vi "ReplaceSelf.vi"(0 "XRef":T9, 1 "Terms":T6, 2 "Diagram":T5, 3 "State In":T4) -> (14 "Replace Self?":T1, 15 "Reply":T2)   [LabVIEW 2012, in "OpenG FilterArray.xnode"]
doc: "This ability VI is called when you want to replace this XNode via LabVIEW's scripting API. This VI is only called when you have previously informed LabVIEW that you want to replace the XNode through a ReplaceSelf reply. Diagram is a reference to a diagram of a temporary VI. This diagram contains exactly one front panel terminal for each terminal of your XNode. Terms is an array of pairs of Term IDs and terminal references. LabVIEW will replace your XNode with code scripted into this diagram into the diagram of the VI containing your XNode and connect everything to the correct terminals. The front panel terminals that are on this diagram are special in that they can only be on the top level diagram.\n \n Replace Self? is used to tell LabVIEW whether or not you want to copy the scripted diagram over. If there is an error and you wish not to commit the changes, then the old XNode behavior will be left unchanged. It will not be called again until you indicate that it should be through the reply on another ability VI.\n \n You should not use the Copy scripting method to move code into the temporary VI. This will adversely affect the user's clipboard. You should use the Move scripting method instead.\n\nDefault behavior: None.\n\nThis ability does not provide UI and OS messages are not handled.\n\nSee also: AugmentSelf"
uses:
  OpenG FilterArray.xnode
  <vilib>/XNodeSupport/XNodeXNodeRef.ctl
  <vilib>/XNodeSupport/XNodeTermIDPairs.ctl
  <vilib>/XNodeSupport/XNodeTermIDPair.ctl
  <vilib>/XNodeSupport/XNodeTermRef.ctl
  <vilib>/XNodeSupport/XNodeString.ctl
  <vilib>/XNodeSupport/XNodeTopLevelDiagramRef.ctl
  State.ctl
  <vilib>/XNodeSupport/XNodeStringArray.ctl
  <vilib>/XNodeSupport/XNodeBool.ctl
  <vilib>/Utility/miscctls.llb/LVPositionTypeDef.ctl
  <userlib>/_LAVAcr/Scripting Tools/Scripting Tools.lvlib
  <vilib>/XNodeSupport/NI_XNodeSupport.lvlib
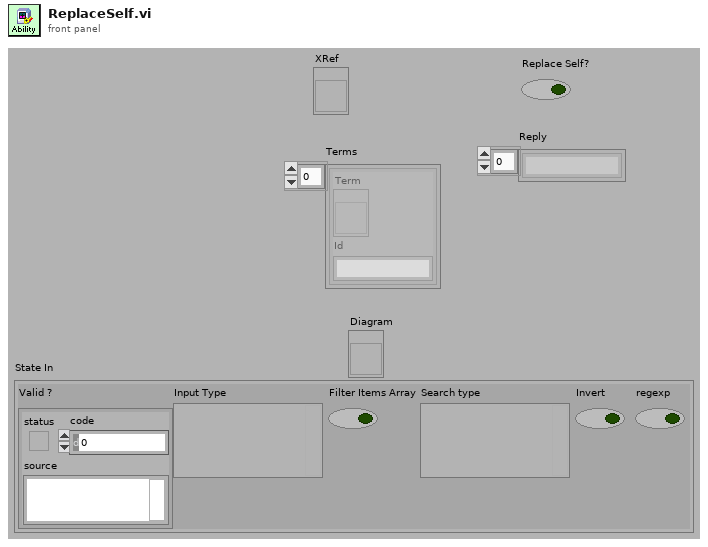
[diagram p1: front panel]
types:
  T1 = typedef "NI_XNodeSupport.lvlib/XNodeBool.ctl" = bool
  T2 = typedef "NI_XNodeSupport.lvlib/XNodeStringArray.ctl" = T3[]
  T3 = typedef "NI_XNodeSupport.lvlib/XNodeString.ctl" = string
  T4 = typedef "OpenG FilterArray.xnode/State.ctl" = cluster{"Valid ?":errorcluster, "Input Type":variant, "Filter Items Array":bool, "Search type":variant, "Invert":bool, "regexp":bool}
  T5 = typedef "NI_XNodeSupport.lvlib/XNodeTopLevelDiagramRef.ctl" = refnum<vi>
  T6 = typedef "NI_XNodeSupport.lvlib/XNodeTermIDPairs.ctl" = T7[]
  T7 = typedef "NI_XNodeSupport.lvlib/XNodeTermIDPair.ctl" = cluster{"Term":T8, "Id":T3}
  T8 = typedef "NI_XNodeSupport.lvlib/XNodeTermRef.ctl" = refnum<vi>
  T9 = typedef "NI_XNodeSupport.lvlib/XNodeXNodeRef.ctl" = refnum<vi>
  T10 = typedef "LVPositionTypeDef.ctl" = cluster{"Left":i32, "Top":i32}
  T11 = typedef "imagedata.ctl" = cluster{"image type":i32, "image depth":i32, "image":u8[], "mask":u8[], "colors":u32[], "Rectangle":cluster{"left":i16, "top":i16, "right":i16, "bottom":i16}}
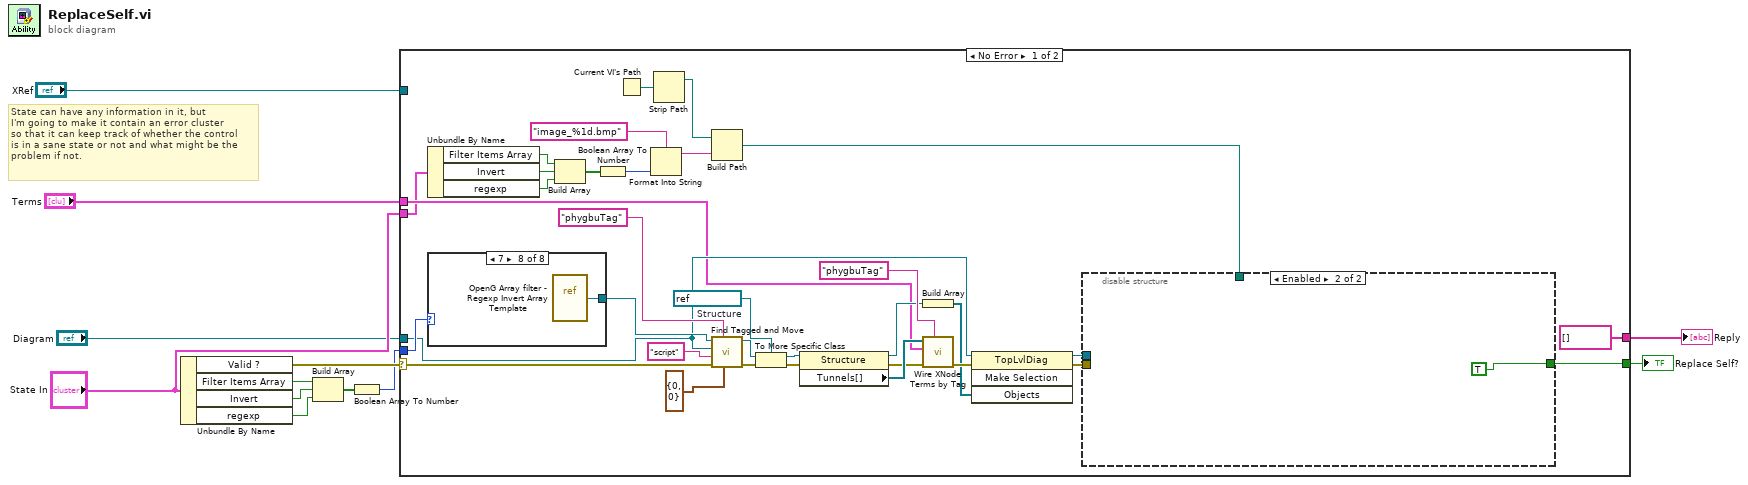
[diagram p0: block diagram]
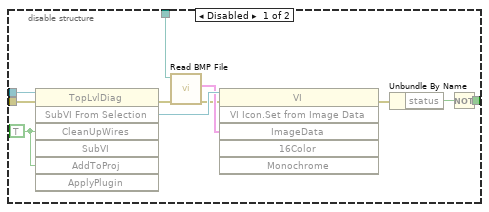
[diagram p2: hidden frame]
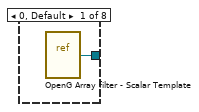
[diagram p3: hidden frame]
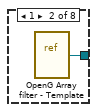
[diagram p4: hidden frame]
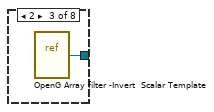
[diagram p5: hidden frame]
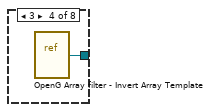
[diagram p6: hidden frame]
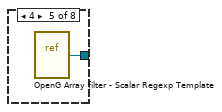
[diagram p7: hidden frame]
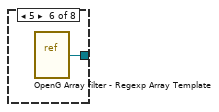
[diagram p8: hidden frame]
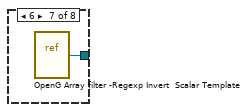
[diagram p9: hidden frame]
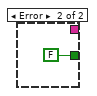
[diagram p10: hidden frame]
diagram:
  # "State can have any information in it, but\nI'm going to make it contain an error cluster\nso that it can keep track of whether the control\nis in a sane state or not and what might be the\nproblem if not."
  n1 = Unbundle By Name("State In") -> ("Valid ?"=w12:errorcluster, "Filter Items Array"=w10:bool, "Invert"=w9:bool, "regexp"=w7:bool)
  n2 = Build Array(w10, w9, w7) -> (w11:bool[])
  n3 = Boolean Array To Number(Boolean array=w11) -> (number=w8:u32)
  n4 = case shown="No Error" w12 {
    selector: w12 -> [w42 _]
    tunnel: "State In" -> [w13 _]
    tunnel: "Diagram" -> [w30 _]
    tunnel: "Terms" -> [w24 _]
    tunnel: [string[] [] ("Reply") _] -> w2
    tunnel: [w31 FALSE] -> w3
    tunnel: w8 -> [w33 _]
    tunnel: "XRef" -> [_ _]
    frame No Error {
      w44 = refnum<vi> refnum  # Structure
      n5 = Unbundle By Name(w13) -> ("Filter Items Array"=w20:bool, "Invert"=w19:bool, "regexp"=w18:bool)
      n6 = case shown="7" w33 {
        tunnel: [w59 w60 w61 w62 w63 w64 w65 w66] -> w32
        frame 0, Default {
          n7 = vi-ref "OpenG Array filter - Scalar Template.vi"() -> (w59:refnum<vi>)
        }
        frame 1 {
          n8 = vi-ref "OpenG Array filter - Template.vi"() -> (w60:refnum<vi>)
        }
        frame 2 {
          n9 = vi-ref "OpenG Array filter -Invert  Scalar Template.vi"() -> (w61:refnum<vi>)
        }
        frame 3 {
          n10 = vi-ref "OpenG Array filter - Invert Array Template.vi"() -> (w62:refnum<vi>)
        }
        frame 4 {
          n11 = vi-ref "OpenG Array filter - Scalar Regexp Template.vi"() -> (w63:refnum<vi>)
        }
        frame 5 {
          n12 = vi-ref "OpenG Array filter - Regexp Array Template.vi"() -> (w64:refnum<vi>)
        }
        frame 6 {
          n13 = vi-ref "OpenG Array filter -Regexp Invert  Scalar Template.vi"() -> (w65:refnum<vi>)
        }
        frame 7 {
          n14 = vi-ref "OpenG Array filter - Regexp Invert Array Template.vi"() -> (w66:refnum<vi>)
        }
      }
      n15 = Build Array(w20, w19, w18) -> (w17:bool[])
      n16 = Boolean Array To Number(Boolean array=w17) -> (number=w15:u32)
      n17 = Current VI's Path() -> (path=w23:path)
      n18 = Format Into String(format string="image_%1d.bmp" ("name or relative path"), w15) -> (resulting string=w14:string)  [unwired: 2 in, 1 out]
      n19 = Strip Path(path=w23) -> (stripped path=w22:path)  [unwired: 1 out]
      n20 = Build Path(base path=w22, name or relative path=w14) -> (appended path=w21:path)
      n21 = call <userlib>:"Find Tagged and Move.vi"("position"=T10 {"Left"=0, "Top"=0}, "TagName"="phygbuTag", "error in"=w42, "TagValue"="script", "Destination Diagram"=w30, "VI Refnum"=w32) -> ("error out"=w37:errorcluster, "Moved Tagged object"=w38:refnum<vi>)  [unwired: 4 out]
      n22 = To More Specific Class(target class=w44, reference=w38, error in=w37) -> (specific class reference=w45:refnum<vi>, error out=w36:errorcluster)
      n23 = property class="Structure"(reference=w45, error in=w36) -> (reference out=w28:refnum<vi>, error out=w35:errorcluster, "Tunnels[]"=w43:refnum<vi>[])
      n24 = Build Array(w28) -> (w27:refnum<vi>[])
      n25 = call <userlib>:"Wire XNode Terms by Tag.vi"("TagName"="phygbuTag", "error in (no error)"=w35, "Term Refs"=w24, "Source References"=w43) -> ("error out"=w29:errorcluster)  [unwired: 7 out]
      n26 = invoke class="TopLvlDiag" method="Make Selection"(reference=w30, error in=w29, "Objects"=w27) -> (reference out=w25:T5, error out=w26:errorcluster)  [unwired: 1 in, 2 out]
      n27 = disable-structure shown="Enabled" {
        disable-tunnel: [w53 TRUE] -> w31
        disable-tunnel: w26 -> [w52 _]
        disable-tunnel: w25 -> [w51 _]
        disable-tunnel: w21 -> [w50 _]
        frame Disabled {
          w57 = TRUE ("Clean Up Wires")
          n28 = invoke class="TopLvlDiag" method="SubVI From Selection"(reference=w51, error in=w52, "CleanUpWires"=w57, "AddToProj"=w57) -> (error out=w48:errorcluster, "SubVIFromSelection"=w56:refnum<vi>)  [unwired: 3 in, 5 out]
          n29 = call <vilib>:"Read BMP File.vi"("error in (no error)"=w48, "path to BMP file"=w50) -> ("error out"=w47:errorcluster, "image data"=w49:T11)  [unwired: 8 out]
          n30 = invoke class="VI" method="VI Icon.Set from Image Data"(reference=w56, error in=w47, "ImageData"=w49) -> (error out=w55:errorcluster)  [unwired: 3 in, 5 out]
          n31 = Unbundle By Name(w55) -> ("status"=w54:bool)
          n32 = Not(x=w54) -> (.not. x?=w53:bool)
        }
        frame Enabled {
        }
      }
    }
    frame Error {
    }
  }
  "Reply" <- w2
  "Replace Self?" <- w3
